vi "EFW Get Position.vi"(8 "error in (no error)":errorcluster caption="错误输入（无错误）", 10 "pPosition":i32, 11 "ID":i32) -> (0 "error out":errorcluster caption="错误输出", 2 "pPosition out":i32, 3 "function return":u32(ring))   [LabVIEW 2012, in "EFW_filter.lvlib"]
doc: "EFW_API EFW_ERROR_CODE EFWGetPosition(int ID, int *pPosition);"
uses:
  <userlib>/EFW_filter/EFW_filter.lvlib
  <userlib>/EFW_filter/EFW_filter.dll
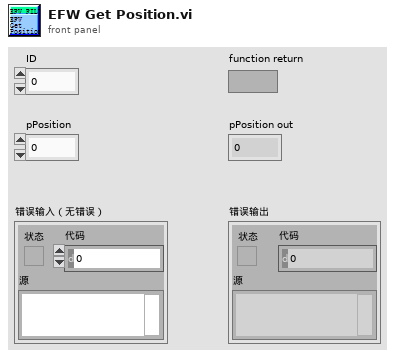
[diagram p1: front panel]
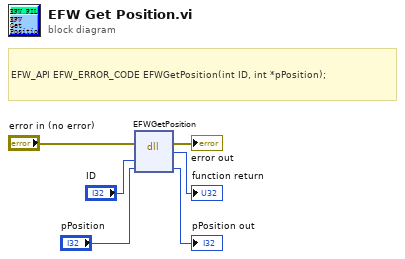
[diagram p0: block diagram]
diagram:
  # "EFW_API\tEFW_ERROR_CODE EFWGetPosition(int ID, int *pPosition);"
  n1 = dll-call lib="D:/Program Files (x86)/National Instruments/LabVIEW 2012/user.lib/EFW_filter/EFW_filter.*" fn="EFWGetPosition"(error in="error in (no error)", "ID"="ID", "pPosition"="pPosition") -> (error out=→"error out":errorcluster, →"function return":u32, "pPosition"=→"pPosition out":i32)  [unwired: 3 in, 1 out]
